vi "Test_PersistToDisk_OneWrite_ValueOK.vi"(8 "error in (no error)":errorcluster, 11 "TestCase in":refnum<class "TestTransport.lvclass">) -> (0 "error out":errorcluster, 3 "TestCase out":refnum<class "TestTransport.lvclass">)   [LabVIEW 2017, in "TestTransport.lvclass"]
uses:
  TestTransport.lvclass
  PersistToDiskTransport/Recovered Value.ctl
  <vilib>/Utility/sysdir.llb/System Directory Type.ctl
  PersistToDiskTransport/PersistToDiskTransport.lvclass/PersistToDiskTransport.ctl
  PersistToDiskTransport/PersistToDiskTransport.lvclass
panel:
  out "Original Value":T1
  out "Recovered Value":T2
  out "Test Folder Path":path
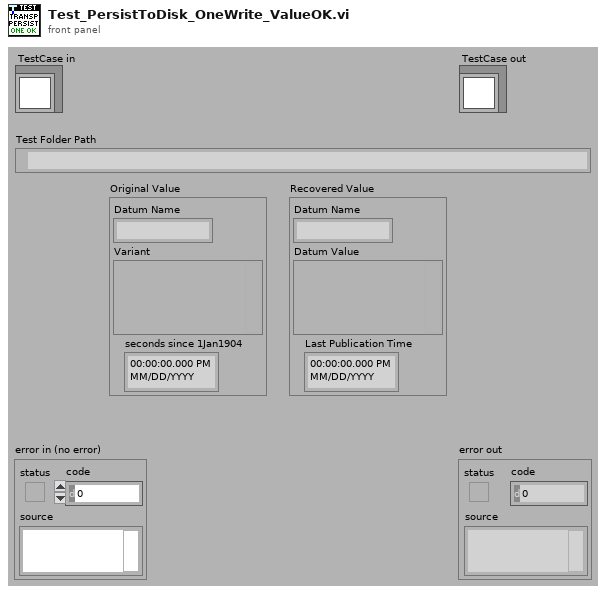
[diagram p1: front panel]
types:
  T1 = cluster{"Datum Name":string, "Variant":variant, "seconds since 1Jan1904":timestamp}
  T2 = typedef "Transport.lvlib/PersistToDiskTransport.lvclass/Recovered Value.ctl" = cluster{"Datum Name":string, "Datum Value":variant, "Last Publication Time":timestamp}
  T3 = typedef "System Directory Type.ctl" = i32
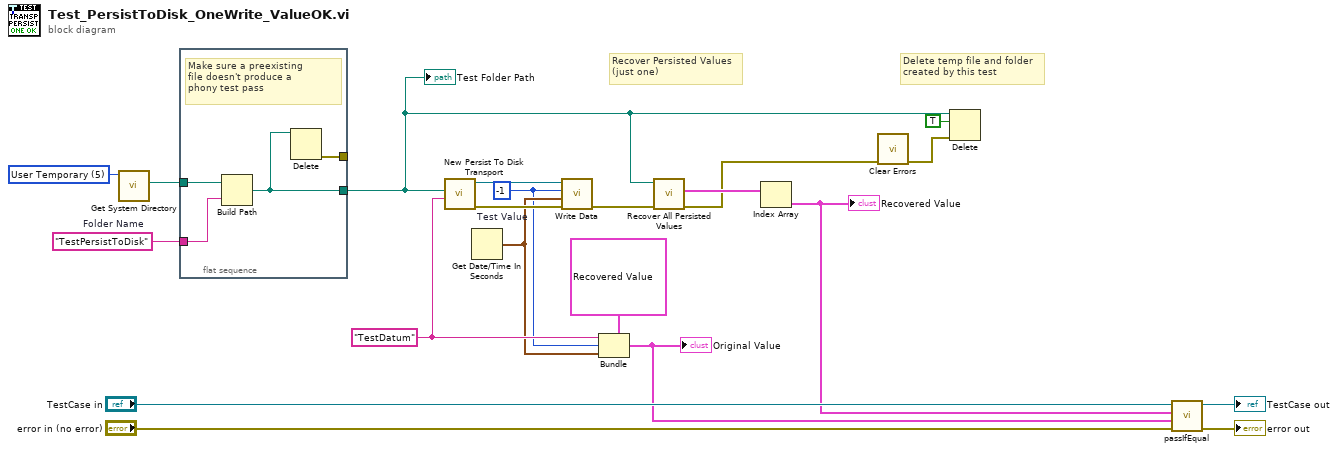
[diagram p0: block diagram]
diagram:
  w11 = "TestDatum" ("Datum Name")
  w9 = -1  # Test Value
  w14 = "TestPersistToDisk"  # Folder Name
  w16 = T3 5 items=["User Home"=0, "User Desktop"=1, "User Documents"=2, "User Application Data"=3, "User Preferences"=4, "User Temporary"=5, "Public Documents"=6, "Public Application Data"=7, "Public Preferences"=8, "Public Cache"=13, "System Core Libraries"=9, "System Installed Libraries"=10, "Application Files"=11, "Boot Volume Root"=12] ("system directory type")
  # "Delete temp file and folder\ncreated by this test"
  # "Recover Persisted Values\n(just one)"
  n1 = call <vilib>:"Get System Directory.vi"("system directory type"=w16) -> ("system directory"=w15:path)  [unwired: 10 in]
  n2 = flat-sequence {
    tunnel: w15 -> [w24]
    tunnel: [w22] -> w5
    tunnel: [w25] -> _
    tunnel: w14 -> [w23]
    frame #0 {
      # "Make sure a preexisting\nfile doesn't produce a\nphony test pass"
      n3 = Build Path(base path=w24, name or relative path=w23) -> (appended path=w22:path)
      n4 = Delete(path (use dialog)=w22) -> (error out=w25:errorcluster)  [unwired: 4 in, 2 out]
    }
  }
  n5 = call "New Persist To Disk Transport.vi"("Datum Name"=w11, "Folder Path"=w5) -> ("error out"=w17:errorcluster, "PersistToDiskTransport Out"=w18:refnum<class "PersistToDiskTransport.lvclass">)  [unwired: 8 in]
  n6 = Get Date/Time In Seconds() -> (seconds since 1Jan1904=w10:timestamp)
  n7 = call-dynamic "Write Data.vi"("error in (no error)"=w17, "Publication Time"=w10, "Value"=w9, "PersistToDiskTransport In"=w18) -> ("error out"=w13:errorcluster)  [unwired: 6 in, 1 out]
  n8 = Bundle(cluster=T2 {"Datum Name"="", "Datum Value"=variant, "Last Publication Time"=timestamp(0 s since 1904-01-01)} ("Recovered Value"), "Datum Name"=w11, "Datum Value"=w9, "Last Publication Time"=w10) -> (w8:T2)
  "Original Value" <- w8
  n9 = call "Recover All Persisted Values.vi"("error in (no error)"=w13, "Folder Path"=w5) -> ("error out"=w4:errorcluster, "Recovered Values"=w12:T2[])  [unwired: 8 in]
  n10 = Index Array(array=w12) -> (element=w7:T2)  [unwired: 1 in]
  "Recovered Value" <- w7
  n11 = call <vilib>:"Clear Errors.vi"("error in (no error)"=w4) -> ("error out"=w3:errorcluster)  [unwired: 5 in, 1 out]
  n12 = Delete(path (use dialog)=w5, entire hierarchy (F)=TRUE, error in=w3) -> ()  [unwired: 2 in, 3 out]
  n13 = call-dynamic "passIfEqual.vi"("error in (no error)"="error in (no error)", "y"=w8, "x"=w7, "TestCase in"="TestCase in") -> ("error out"=→"error out":errorcluster, "TestCase out"=→"TestCase out":refnum<class "TestTransport.lvclass">)  [unwired: 6 in]
  "Test Folder Path" <- w5
